vi "Get Target Custom Devices (SubVI).vi"(8 "error in (no error)":errorcluster, 11 "Target Refnum in":refnum<k24>) -> (0 "error out":errorcluster, 1 "CD Names out":string[](array[string]), 2 "Custom Devices Refnums":refnum<k24>[](array[refnum]), 3 "Target Refnum out":refnum<k24>)   [LabVIEW 2020, in "FPGA Addon Test Class.lvclass"]
uses:
  FPGA Addon Test Class.lvclass
  NationalInstruments.VeriStand.SystemDefinitionAPI
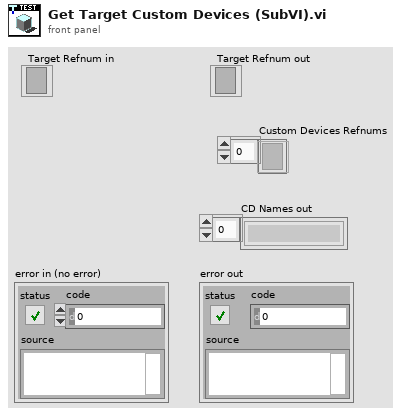
[diagram p1: front panel]
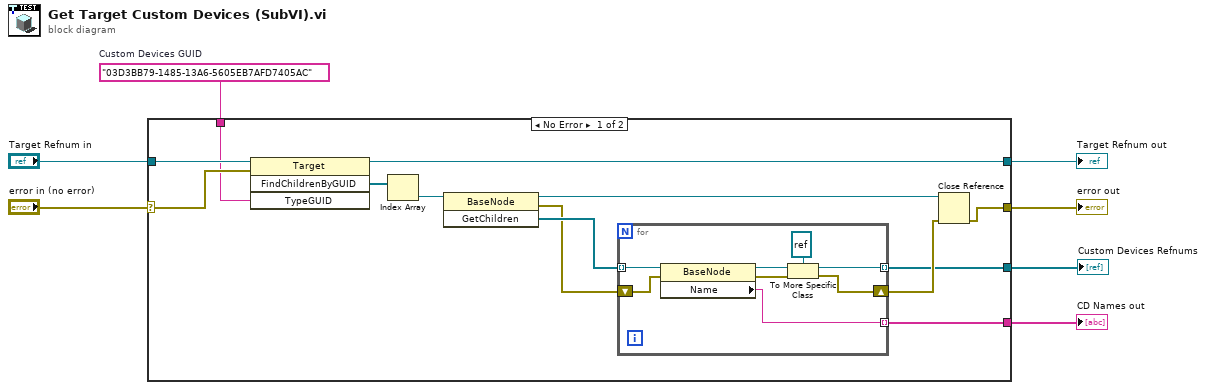
[diagram p0: block diagram]
diagram:
  w3 = "03D3BB79-1485-13A6-5605EB7AFD7405AC"  # Custom Devices GUID
  n1 = case shown="No Error" "error in (no error)" {
    selector: "error in (no error)" -> [w19 w30]
    tunnel: [w10 w30] -> w6
    tunnel: "Target Refnum in" -> [w20 w29]
    tunnel: [w16 w29] -> w2
    tunnel: w3 -> [w18 _]
    tunnel: [w9 _] -> w7
    tunnel: [w8 _] -> w1
    frame No Error {
      n2 = invoke class="Target" method="FindChildrenByGUID"(reference=w20, error in=w19, "TypeGUID"=w18) -> (reference out=w16:refnum<k24>, "FindChildrenByGUID"=w17:refnum<k24>[])  [unwired: 1 in, 2 out]
      n3 = Index Array(array=w17) -> (element=w15:refnum<k24>)  [unwired: 1 in]
      n4 = invoke class="BaseNode" method="GetChildren"(reference=w15) -> (reference out=w14:refnum<k24>, error out=w12:errorcluster, "GetChildren"=w13:refnum<k24>[])  [unwired: 2 in]
      n5 = for {
        tunnel: w13 -> [w28] mode=indexing
        shift-right: [w23] -> w11
        shift-left: w12 -> [w27]
        tunnel: [w26] -> w9 mode=indexing
        tunnel: [w22] -> w8 mode=indexing
        n6 = property class="BaseNode"(reference=w28, error in=w27) -> (reference out=w25:refnum<k24>, error out=w24:errorcluster, "Name"=w26:string)
        n7 = To More Specific Class(target class=refnum<k24> refnum ("new reference"), reference=w25, error in=w24) -> (specific class reference=w22:refnum<k24>, error out=w23:errorcluster)
      }
      n8 = Close Reference(reference=w14, error in (no error)=w11) -> (error out=w10:errorcluster)
    }
    frame Error {
    }
  }
  "CD Names out" <- w7
  "error out" <- w6
  "Target Refnum out" <- w2
  "Custom Devices Refnums" <- w1
